vi "Water Cooled Simulator.vi"() -> ()   [LabVIEW 2026]
uses:
  Turbine Build Specifications.ctl
  Fission Reactor Build Specifications.ctl
  Induction Matrix Build Specifications.ctl
  Port Defs/Reactor Port States.ctl
  Port Defs/Turbine Port States.ctl
  Port Defs/Matrix Port States.ctl
  Tier.ctl
panel:
  in  "Reactor Port States":T1={"Cooled Coolant (mB/t)"=0, "Waste (mB/t)"=0, "Heated Coolant (mB/t)"=1000000}
  out "Waste (mB)":i64
  in  "Biome Temperature":dbl=0.9 format="%#_13g"
  out "TPS":dbl
  out "Tick Duration":u32
  in  "Matrix Build Specifications":T2={"Length (m)"=3, "Width (m)"=3, "Height (m)"=4, "Matrix Blocks"={"Basic Cells"=0, "Advanced Cells"=0, "Elite Cells"=0, "Ultimate Cells"=0, "Basic Providers"=0, "Advanced Providers"=0, "Elite Providers"=0, "Ultimate Providers"=0}} {"Height (m)" min=3 max=18 step=1; "Width (m)" min=3 max=18 step=1; "Length (m)" min=3 max=18 step=1}
  in  "Reactor Build Specifications":T3={"Length (m)"=3, "Width (m)"=3, "Height (m)"=4, "Coolant Type"=enum."Water"} {"Height (m)" min=4 max=18 step=1; "Width (m)" min=3 max=18 step=1; "Length (m)" min=3 max=18 step=1}
  in  "Turbine Build Specifications":T4={"Length (m)"=17, "Width (m)"=17, "Height (m)"=18, "Condenser Layers"=1, "Rotor Height"=14, "Vents"=345, "Condensers"=218} {"Condensers" min=0 step=1; "Vents" min=0 step=1; "Rotor Height" min=0 max=14 step=1; "Condenser Layers" min=0 max=14 step=1; "Height (m)" min=4 max=18 step=1; "Width (m)" min=5 max=17 step=2; "Length (m)" min=5 max=17 step=2}
  out "Temperature (K)":dbl
  out "Heating Rate (mB/t)":i64
  in  "Fuel Input (mB/t)":i64
  in  "Activate":bool
  in  "Burn Rate (mB/t)":dbl min=0.0 max=1.0
  in  "stop":bool
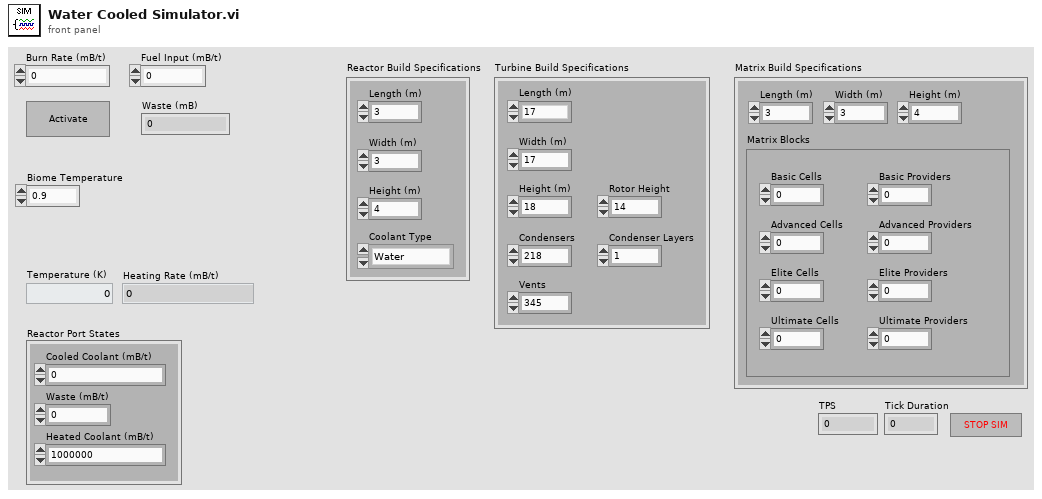
[diagram p1: front panel]
types:
  T1 = typedef "Reactor Port States.ctl" = cluster{"Cooled Coolant (mB/t)":i64, "Waste (mB/t)":i64, "Heated Coolant (mB/t)":i64}
  T2 = typedef "Induction Matrix Build Specifications.ctl" = cluster{"Length (m)":i32, "Width (m)":i32, "Height (m)":i32, "Matrix Blocks":cluster{"Basic Cells":u64, "Advanced Cells":u64, "Elite Cells":u64, "Ultimate Cells":u64, "Basic Providers":u64, "Advanced Providers":u64, "Elite Providers":u64, "Ultimate Providers":u64}}
  T3 = typedef "Fission Reactor Build Specifications.ctl" = cluster{"Length (m)":i32, "Width (m)":i32, "Height (m)":i32, "Coolant Type":enum16{"Water", "Sodium"}}
  T4 = typedef "Turbine Build Specifications.ctl" = cluster{"Length (m)":i32, "Width (m)":i32, "Height (m)":i32, "Condenser Layers":i32, "Rotor Height":i32, "Vents":i32, "Condensers":i32}
  T5 = typedef "Matrix Port States.ctl" = cluster{"Energy (FE)":ext}
  T6 = typedef "Turbine Port States.ctl" = cluster{"Steam (mB/t)":i64, "Water (mB/t)":i64, "Energy (FE)":ext}
  T7 = typedef "Tier.ctl" = enum16{"BASIC", "ADVANCED", "ELITE", "ULTIMATE"}
  T8 = cluster{"Tier":T7, "Acceptors":i64, "Length":i64, "Transmitters":i64}
  T9 = typedef "Fission Reactor Build Properties.ctl" = cluster{"Fuel Rods":i32, "Control Rods":i32, "Volume (m³)":i32, "Fuel Surface Area (m²)":i32, "Cooled Coolant Tank (mB)":i32, "Fuel Capacity (mB)":i64, "Heat Capacity (J/K)":dbl, "Max Burn Rate":i64, "Max Heating Rate (mB/t)":i64, "Boil Efficiency":dbl, "Coolant Type":enum16{"Water", "Sodium"}, "Heated Coolant Tank (mB)":i64}
  T10 = typedef "Induction Matrix Build Properties.ctl" = cluster{"Internal Volume (m³)":i32, "Volume (m³)":i32, "Storage (FE)":ext, "Provider Rate (FE/t)":ext}
  T11 = typedef "Turbine Build Properties.ctl" = cluster{"Volume (m³)":i32, "Rotor Height (m)":i32, "Condensers":i32, "Vents":i32, "Rotor Blades":i32, "Coils":i32, "Dispersers":i32, "Steam Tank (mB)":i64, "Energy Capacity (FE)":ext, "Vent Flow Rate (mB/t)":dbl, "Max Water Return (mB/t)":i32, "Area (m²)":i32, "Inner Area (m²)":i32}
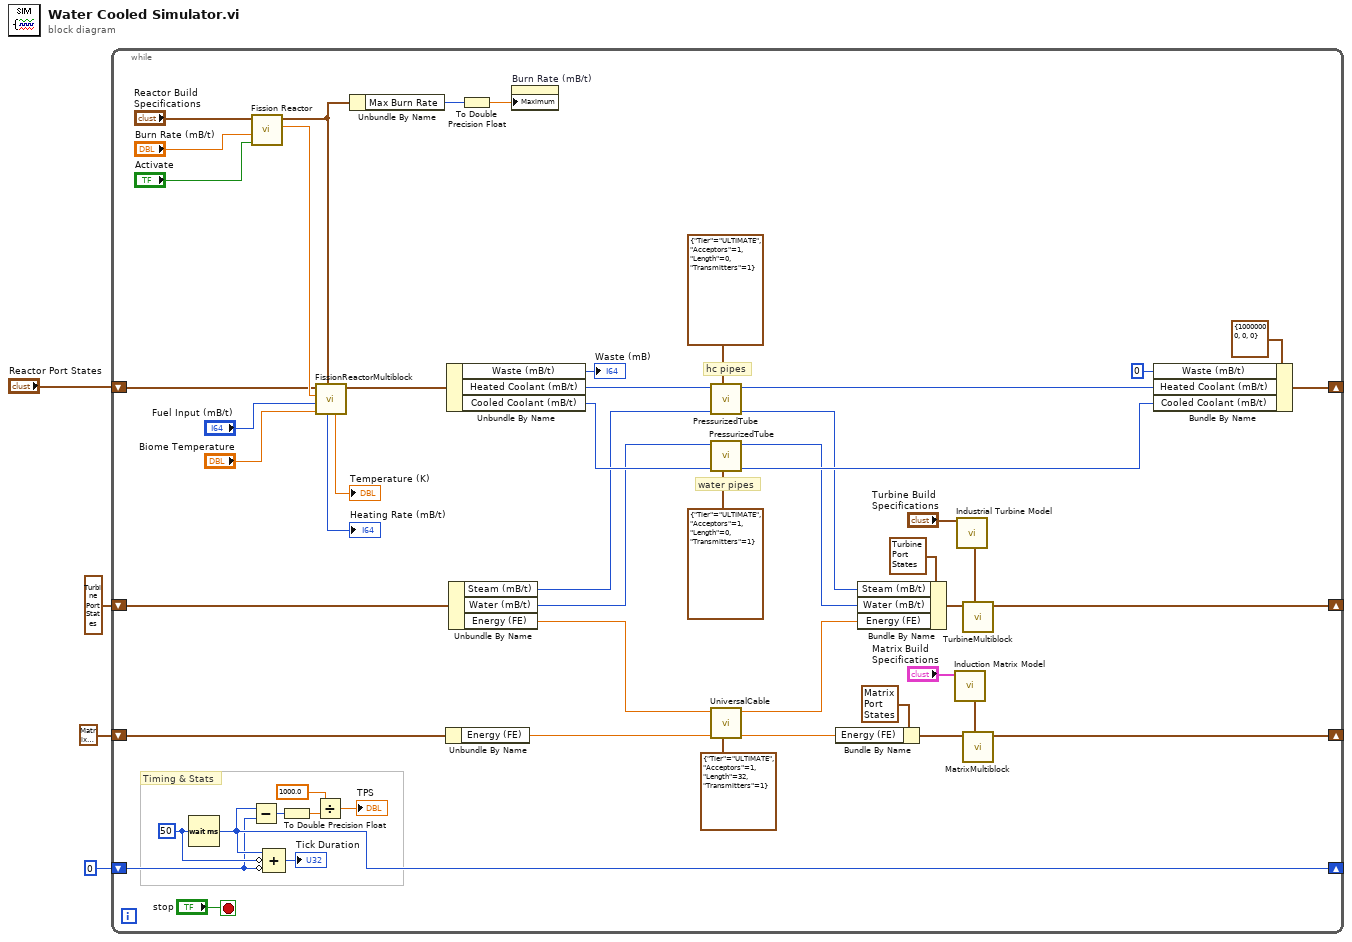
[diagram p0: block diagram]
diagram:
  n1 = while {
    shift-right: [w34] -> _
    shift-left: "Reactor Port States" -> [w27]
    shift-right: [w40] -> _
    shift-left: u32 0 ("millisecond timer value") -> [w39]
    shift-right: [w23] -> _
    shift-left: T6 {"Steam (mB/t)"=0, "Water (mB/t)"=0, "Energy (FE)"=0.0} ("Port States Out") -> [w22]
    shift-right: [w13] -> _
    shift-left: T5 {"Energy (FE)"=0.0} ("Induction Matrix Port States") -> [w10]
    stop <- "stop" stop-if-true
    w41 = u32 50 ("milliseconds to wait")
    # "hc pipes"
    # "water pipes"
    # "Timing & Stats"
    n2 = Wait (ms)(milliseconds to wait=w41) -> (millisecond timer value=w40:u32)
    n3 = Subtract(x=w40, y=w39) -> (x-y=w38:u32)
    n4 = call "Fission Reactor.vi"("Activate"="Activate", "Burn Rate (mB/t)"="Burn Rate (mB/t)", "Build Specifications"="Reactor Build Specifications") -> ("Actual Burn Rate (mB/t)"=w32:dbl, "Computed Build Properties"=w50:T9)  [unwired: 6 in, 1 out]
    n5 = Compound Arithmetic op=ADD(w40, invert w41, invert w39) -> (→"Tick Duration":u32)
    n6 = To Double Precision Float(number=w38) -> (double precision float=w35:dbl)
    n7 = Divide(x=1000.0 ("y"), y=w35) -> (x/y=→"TPS":dbl)
    n8 = call "FissionReactorMultiblock.vi"("Reactor Build Properties"=w50, "Biome Temperature"="Biome Temperature", "Fuel Input (mB/t)"="Fuel Input (mB/t)", "Burn Rate (mB/t)"=w32, "Port States In"=w27) -> ("Port States Out"=w31:T1, "Temperature (K)"=→"Temperature (K)":dbl, "Heating Rate (mB/t)"=→"Heating Rate (mB/t)":i64)  [unwired: 4 in]
    n9 = Unbundle By Name(w50) -> ("Max Burn Rate"=w54:i64)
    n10 = Unbundle By Name(w10) -> ("Energy (FE)"=w6:ext)
    n11 = Unbundle By Name(w31) -> ("Waste (mB/t)"=→"Waste (mB)":i64, "Heated Coolant (mB/t)"=w18:i64, "Cooled Coolant (mB/t)"=w56:i64)
    n12 = Unbundle By Name(w22) -> ("Steam (mB/t)"=w21:i64, "Water (mB/t)"=w16:i64, "Energy (FE)"=w9:ext)
    n13 = To Double Precision Float(number=w54) -> (double precision float=w53:dbl)
    n14 = property on="Burn Rate (mB/t)" class="DigNum (strict)"("Maximum"=w53) -> ()  [unwired: 2 in, 2 out]
    n15 = call "PressurizedTube.vi"("Pipe Network Parameters"=T8 {"Tier"=enum."ULTIMATE", "Acceptors"=1, "Length"=0, "Transmitters"=1}, "Unused Output (mB/t)"=w21, "Push Input (mB/t)"=w18) -> ("Output (mB/t)"=w17:i64, "Rejected Input (mB/t)"=w19:i64)  [unwired: 5 in, 2 out]
    n16 = call "PressurizedTube.vi"("Pipe Network Parameters"=T8 {"Tier"=enum."ULTIMATE", "Acceptors"=1, "Length"=0, "Transmitters"=1}, "Unused Output (mB/t)"=w56, "Push Input (mB/t)"=w16) -> ("Output (mB/t)"=w57:i64, "Rejected Input (mB/t)"=w15:i64)  [unwired: 5 in, 2 out]
    n17 = call "UniversalCable.vi"("Cable Network Parameters"=T8 {"Tier"=enum."ULTIMATE", "Acceptors"=1, "Length"=32, "Transmitters"=1}, "Unused Output (FE/t)"=w6, "Push Input (FE/t)"=w9) -> ("Output (FE/t)"=w7:ext, "Rejected Input (FE/t)"=w8:ext)  [unwired: 5 in, 2 out]
    n18 = Bundle By Name(cluster=T5 {"Energy (FE)"=0.0} ("Induction Matrix Port States"), "Energy (FE)"=w7) -> (w11:T5)
    n19 = Bundle By Name(cluster=T6 {"Steam (mB/t)"=0, "Water (mB/t)"=0, "Energy (FE)"=0.0} ("Port States In"), "Steam (mB/t)"=w17, "Water (mB/t)"=w15, "Energy (FE)"=w8) -> (w30:T6)
    n20 = call "Induction Matrix Model.vi"("Build Specifications"="Matrix Build Specifications") -> ("Induction Matrix Build Properties"=w48:T10)  [unwired: 6 in, 4 out]
    n21 = call "Industrial Turbine Model.vi"("Turbine Build Specifications"="Turbine Build Specifications") -> ("Turbine Build Properties"=w49:T11)  [unwired: 10 in, 8 out]
    n22 = call "TurbineMultiblock.vi"("Turbine Build Properties"=w49, "Port States In"=w30) -> ("Port States Out"=w23:T6)  [unwired: 9 in]
    n23 = call "MatrixMultiblock.vi"("Induction Matrix Build Properties"=w48, "Port States In"=w11) -> ("Port States Out"=w13:T5)  [unwired: 9 in]
    n24 = Bundle By Name(cluster=T1 {"Cooled Coolant (mB/t)"=10000000, "Waste (mB/t)"=0, "Heated Coolant (mB/t)"=0} ("Reactor Port States"), "Waste (mB/t)"=i64 0, "Heated Coolant (mB/t)"=w19, "Cooled Coolant (mB/t)"=w57) -> (w34:T1)
  }
